vi "kuup2evKell.vi"(6 "Sisend":string[](array[string]), 7 "Kuni (kellaaeg)":string, 8 "Kuni (kuupäev)":string, 9 "Alates (kellaaeg)":string, 10 "Alates (kuupäev)":string) -> (3 "V2ljund":string[](array[string]))   [LabVIEW 2012]
panel:
  out "alates":i32
  out "concatenated string 2":string
  out "kuni":i32
  out "concatenated string":string
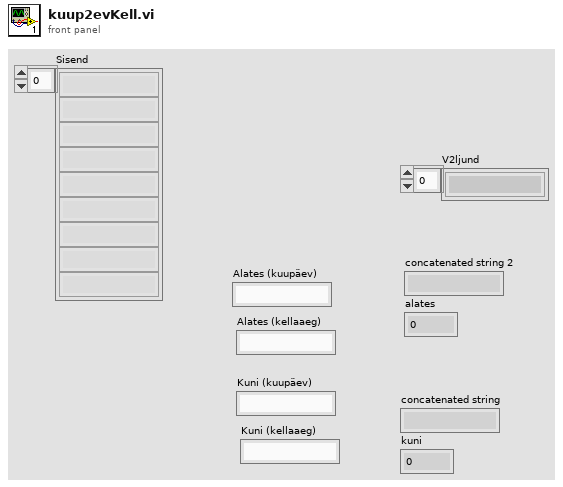
[diagram p1: front panel]
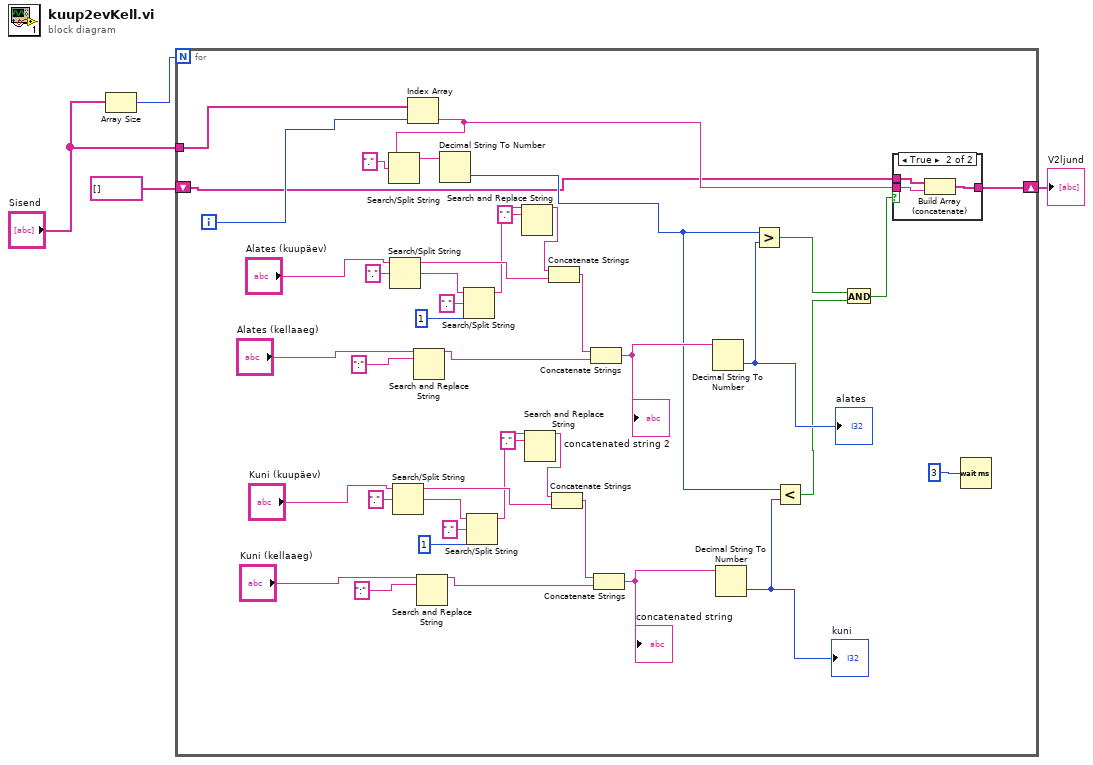
[diagram p0: block diagram]
diagram:
  n1 = Array Size(array="Sisend") -> (size(s)=w4:i32)
  n2 = for {
    N: w4 -> [_]
    shift-right: [w14] -> w3
    shift-left: string[] [] -> [w6]
    tunnel: "Sisend" -> [w5]
    i -> [w15]
    n3 = Search/Split String(string="Alates (kuupäev)", search string/char (-)=".") -> (substring before match=w24:string, match + rest of string=w25:string)  [unwired: 1 in, 1 out]
    n4 = Search/Split String(string="Kuni (kuupäev)", search string/char (-)=".") -> (substring before match=w38:string, match + rest of string=w39:string)  [unwired: 1 in, 1 out]
    n5 = Index Array(array=w5, index=w15) -> (element=w16:string)
    n6 = Search/Split String(string=w16, search string/char (-)=".") -> (substring before match=w17:string)  [unwired: 1 in, 2 out]
    n7 = Search and Replace String(input string="Alates (kellaaeg)", search string=":") -> (result string=w29:string)  [unwired: 6 in, 3 out]
    n8 = Search and Replace String(input string="Kuni (kellaaeg)", search string=":") -> (result string=w43:string)  [unwired: 6 in, 3 out]
    n9 = Decimal String To Number(string=w17) -> (number=w11:i32)  [unwired: 2 in, 1 out]
    n10 = Search/Split String(string=w25, search string/char (-)=".", offset (0)=1) -> (substring before match=w22:string)  [unwired: 2 out]
    n11 = Search/Split String(string=w39, search string/char (-)=".", offset (0)=1) -> (substring before match=w36:string)  [unwired: 2 out]
    n12 = Search and Replace String(input string=w22, search string=".") -> (result string=w20:string)  [unwired: 6 in, 3 out]
    n13 = Search and Replace String(input string=w36, search string=".") -> (result string=w34:string)  [unwired: 6 in, 3 out]
    n14 = Concatenate Strings(w20, w24) -> (w23:string)
    n15 = Concatenate Strings(w34, w38) -> (w37:string)
    n16 = Concatenate Strings(w23, w29) -> (w19:string)
    "concatenated string 2" <- w19
    n17 = Concatenate Strings(w37, w43) -> (w33:string)
    "concatenated string" <- w33
    n18 = Decimal String To Number(string=w19) -> (number=w12:i32)  [unwired: 2 in, 1 out]
    "alates" <- w12
    n19 = Decimal String To Number(string=w33) -> (number=w10:i32)  [unwired: 2 in, 1 out]
    "kuni" <- w10
    n20 = Greater?(x=w11, y=w12) -> (0:w13:bool)
    n21 = Less?(x=w11, y=w10) -> (x < y?=w9:bool)
    n22 = And(x=w13, y=w9) -> (x .and. y?=w8:bool)
    n23 = case shown="True" w8 {
      tunnel: w16 -> [_ w50]
      tunnel: [w47 w49] -> w14
      tunnel: w6 -> [w47 w48]
      frame False {
      }
      frame True {
        n24 = Build Array (concatenate)(w48, w50) -> (w49:string[])
      }
    }
    n25 = Wait (ms)(milliseconds to wait=u32 3 ("delay kuupäev")) -> ()  [unwired: 1 out]
  }
  "V2ljund" <- w3
